vi "Write Color.vi"(9 "color":T1, 11 "Circle":T2) -> (3 "Circle 2":T2)   [LabVIEW 2015, in "Circle Library.lvlib"]
uses:
  Circle Library.lvlib
  Circle cluster.ctl
  colors.ctl
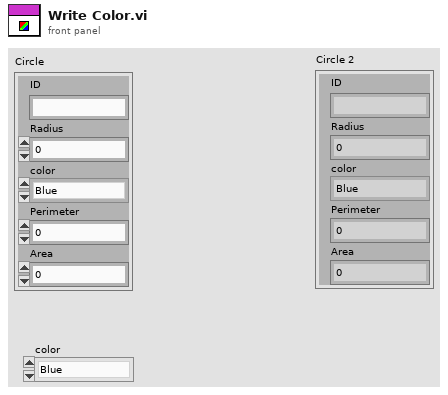
[diagram p1: front panel]
types:
  T1 = typedef "colors.ctl" = enum16{"Blue", "Red", "Green", "Yellow"}
  T2 = typedef "Circle Library.lvlib/Circle cluster.ctl" = cluster{"ID":string, "Radius":dbl, "color":T1, "Perimeter":dbl, "Area":dbl}
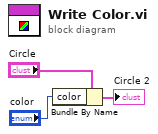
[diagram p0: block diagram]
diagram:
  n1 = Bundle By Name(cluster="Circle", "color"="color") -> (→"Circle 2":T2)
